vi "Manage Robot Shape.vi"(4 "Lighter":bool, 6 "Coords":cluster{"x":dbl, "y":dbl}, 7 "Drawing Options":T1, 8 "Operation":enum16{"Draw", "Pt Test"}(ring), 9 "new picture in":picture, 10 "Robot Position (ft)":cluster{"x":dbl, "y":dbl, "th":dbl}, 11 "Pict Ref":refnum<vi>) -> (0 "Pt Test Results":enum16{"Miss", "Rect Hit", "Arrow Hit"}(ring), 1 "new picture out":picture, 2 "Boundary Poly":cluster{dbl, dbl}[](array[cluster]))   [LabVIEW 2019]
uses:
  <vilib>/Analysis/geometry.llb/Point in Polygon Position.ctl
  Globals.vi
  <vilib>/Analysis/geometry.llb/Point in Polygon (Scalar).vi
  <vilib>/Analysis/NI_AAL_Geometry.lvlib
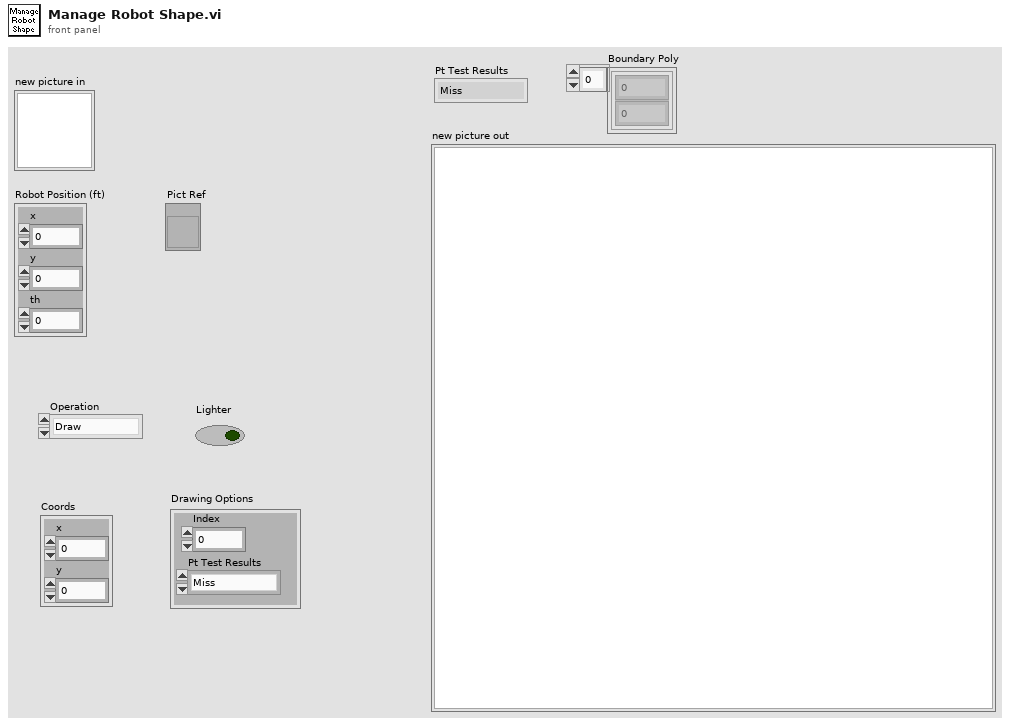
[diagram p1: front panel]
types:
  T1 = cluster{"Index":u32, "Pt Test Results":enum16{"Miss", "Rect Hit", "Arrow Hit"}}
  T2 = typedef "LVPositionTypeDef.ctl" = cluster{"Left":i32, "Top":i32}
  T3 = typedef "LVBoundsTypeDef.ctl" = cluster{"Width":u32, "Height":u32}
  T4 = cluster{"Width":u16, "Style":enum32{"Solid", "Dash", "Dot", "DashDot", "DashDotDot"}}
  T5 = typedef "NI_AAL_Geometry.lvlib/Point in Polygon Position.ctl" = u16
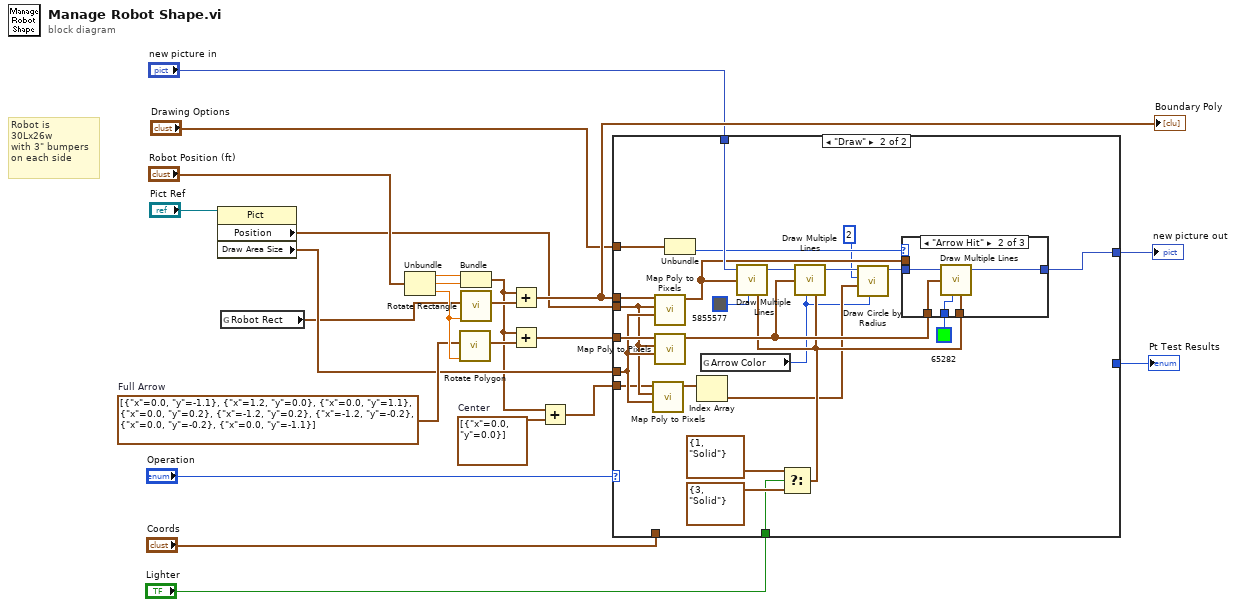
[diagram p0: block diagram]
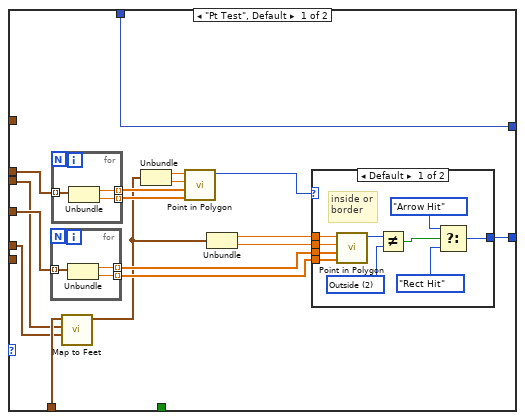
[diagram p2: hidden frame]
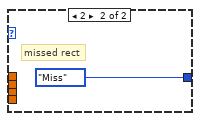
[diagram p3: hidden frame]
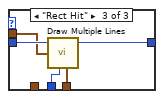
[diagram p5: hidden frame]
diagram:
  w4 = cluster{"x":dbl, "y":dbl}[] [{"x"=0.0, "y"=0.0}]  # Center
  w13 = cluster{"x":dbl, "y":dbl}[] [{"x"=0.0, "y"=-1.1}, {"x"=1.2, "y"=0.0}, {"x"=0.0, "y"=1.1}, {"x"=0.0, "y"=0.2}, {"x"=-1.2, "y"=0.2}, {"x"=-1.2, "y"=-0.2}, {"x"=0.0, "y"=-0.2}, {"x"=0.0, "y"=-1.1}]  # Full Arrow
  # "Robot is\n30Lx26w\nwith 3\" bumpers\non each side"
  n1 = property on="Property Node" class="Pict"(reference="Pict Ref") -> ("Position"=w12:T2, "Draw Area Size"=w11:T3)  [unwired: 1 in, 2 out]
  n2 = global read "Globals.vi" "Robot Rect"() -> (w1:cluster{"x":dbl, "y":dbl, "x":dbl, "y":dbl})
  n3 = Unbundle("Robot Position (ft)") -> ("x"=w15:dbl, "y"=w16:dbl, "th"=w18:dbl)
  n4 = call "Rotate Polygon.vi"("Angle"=w18, "polygon 2"=w13) -> ("polygon"=w22:cluster{dbl, dbl}[])  [unwired: 9 in]
  n5 = Bundle("x"=w15, "y"=w16) -> (w3:cluster{"x":dbl, "y":dbl})  [unwired: 1 in]
  n6 = call "Rotate Rectangle.vi"("Angle"=w18, "Rectangle"=w1) -> ("polygon"=w21:cluster{dbl, dbl}[])  [unwired: 9 in]
  n7 = Add(x=w3, y=w21) -> (x+y=w20:cluster{dbl, dbl}[])
  "Boundary Poly" <- w20
  n8 = Add(x=w3, y=w22) -> (x+y=w23:cluster{dbl, dbl}[])
  n9 = Add(x=w3, y=w4) -> (x+y=w2:cluster{"x":dbl, "y":dbl}[])
  n10 = case shown="\"Draw\"" "Operation" {
    tunnel: w23 -> [w34 w81]
    tunnel: w20 -> [w36 w80]
    tunnel: [w35 w77] -> w19
    tunnel: "new picture in" -> [w35 w78]
    tunnel: w12 -> [w24 w62]
    tunnel: w11 -> [w25 w63]
    tunnel: "Coords" -> [w26 _]
    tunnel: [w28 _] -> w7
    tunnel: "Drawing Options" -> [_ w74]
    tunnel: "Lighter" -> [_ w69]
    tunnel: w2 -> [_ w61]
    frame "Pt Test", Default {
      n11 = for {
        tunnel: w34 -> [w54] mode=indexing
        tunnel: [w53] -> w30 mode=indexing
        tunnel: [w52] -> w29 mode=indexing
        n12 = Unbundle(w54) -> (w53:dbl, w52:dbl)
      }
      n13 = for {
        tunnel: w36 -> [w57] mode=indexing
        tunnel: [w56] -> w39 mode=indexing
        tunnel: [w55] -> w40 mode=indexing
        n14 = Unbundle(w57) -> (w56:dbl, w55:dbl)
      }
      n15 = call "Map to Feet.vi"("Draw Area Size"=w25, "Position"=w24, "Coords (px)"=w26) -> ("Point (ft)"=w27:cluster{dbl, dbl})  [unwired: 8 in]
      n16 = Unbundle(w27) -> (w38:dbl, w37:dbl)
      n17 = call-poly <vilib>:"Point in Polygon.vi"("Polygon Y"=w40, "Polygon X"=w39, "y"=w37, "x"=w38) -> ("position"=w33:T5)  [unwired: 6 in, 1 out]
      n18 = Unbundle(w27) -> (w32:dbl, w31:dbl)
      n19 = case shown="Default" w33 {
        tunnel: w32 -> [w50 _]
        tunnel: w31 -> [w49 _]
        tunnel: w30 -> [w48 _]
        tunnel: w29 -> [w47 _]
        tunnel: [w42 enum16{"Miss", "Rect Hit", "Arrow Hit"}."Miss" ("Pt Test Results")] -> w28
        frame Default {
          w46 = T5 2 items=["Inside", "On Boundary", "Outside"] ("position")
          # "inside or\nborder"
          n20 = call-poly <vilib>:"Point in Polygon.vi"("Polygon Y"=w47, "Polygon X"=w48, "y"=w49, "x"=w50) -> ("position"=w45:T5)  [unwired: 6 in, 1 out]
          n21 = Not Equal?(x=w45, y=w46) -> (x != y?=w41:bool)
          n22 = Select(t=enum16{"Miss", "Rect Hit", "Arrow Hit"}."Arrow Hit" ("Pt Test Results"), s=w41, f=enum16{"Miss", "Rect Hit", "Arrow Hit"}."Rect Hit" ("Pt Test Results")) -> (s? t:f=w42:enum16{"Miss", "Rect Hit", "Arrow Hit"})
        }
        frame 2 {
          # "missed rect"
        }
      }
    }
    frame "Draw" {
      n23 = call "Map Poly to Pixels.vi"("Draw Area Size"=w63, "Position"=w62, "Coords"=w61) -> ("Coords"=w60:cluster{"Horizontal":dbl, "Vertical":dbl}[])  [unwired: 8 in]
      n24 = call "Map Poly to Pixels.vi"("Draw Area Size"=w63, "Position"=w62, "Coords"=w80) -> ("Coords"=w73:cluster{"Horizontal":dbl, "Vertical":dbl}[])  [unwired: 8 in]
      n25 = call "Map Poly to Pixels.vi"("Draw Area Size"=w63, "Position"=w62, "Coords"=w81) -> ("Coords"=w76:cluster{"Horizontal":dbl, "Vertical":dbl}[])  [unwired: 8 in]
      n26 = Unbundle(w74) -> ("Pt Test Results"=w72:enum16{"Miss", "Rect Hit", "Arrow Hit"})  [unwired: 1 out]
      n27 = Index Array(array=w60) -> (element=w59:cluster{"Horizontal":dbl, "Vertical":dbl})  [unwired: 1 in]
      n28 = global read "Globals.vi" "Arrow Color"() -> (w58:u32)
      n29 = Select(t=T4 {"Width"=1, "Style"=enum."Solid"} ("pen"), s=w69, f=T4 {"Width"=3, "Style"=enum."Solid"} ("pen")) -> (s? t:f=w68:T4)
      n30 = call <vilib>:"Draw Multiple Lines.vi"("picture"=w78, "line endpoints"=w73, "color(black)"=u32 5855577, "pen"=w68) -> ("new picture"=w79:picture)  [unwired: 5 in]
      n31 = call <vilib>:"Draw Multiple Lines.vi"("picture"=w79, "line endpoints"=w76, "color(black)"=w58, "pen"=w68) -> ("new picture"=w66:picture)  [unwired: 5 in]
      n32 = call <vilib>:"Draw Circle by Radius.vi"("color(black)"=w58, "pixel center"=w59, "radius"=i16 2, "picture"=w66) -> ("new picture"=w65:picture)  [unwired: 7 in]
      n33 = case shown="\"Arrow Hit\"" w72 {
        tunnel: w65 -> [w82 w87 w92]
        tunnel: [w82 w86 w91] -> w77
        tunnel: w76 -> [_ w85 _]
        tunnel: u32 65282 ("color(black)") -> [_ w84 w90]
        tunnel: w73 -> [_ _ w89]
        tunnel: w68 -> [_ w83 w88]
        frame Default {
        }
        frame "Arrow Hit" {
          n34 = call <vilib>:"Draw Multiple Lines.vi"("picture"=w87, "line endpoints"=w85, "color(black)"=w84, "pen"=w83) -> ("new picture"=w86:picture)  [unwired: 5 in]
        }
        frame "Rect Hit" {
          n35 = call <vilib>:"Draw Multiple Lines.vi"("picture"=w92, "line endpoints"=w89, "color(black)"=w90, "pen"=w88) -> ("new picture"=w91:picture)  [unwired: 5 in]
        }
      }
    }
  }
  "new picture out" <- w19
  "Pt Test Results" <- w7
